vi "Top Menu.vi"(11 "Menu Queue":refnum<queue>) -> ()   [LabVIEW 2013, in "main.lvlib"]
uses:
  main.lvlib
  Controls/Reference AE Control.ctl
  Controls/Reference Cluster.ctl
panel:
  in  "Journal":bool
  in  "Data":bool
  in  "Acquisition":bool
  in  "Configuration":bool
  in  "Profile":bool
  out "PersonalInfoString":string caption="PersonalInfoString2"
  in  "Stop Acq":bool caption="Stop acq"
  in  "MenuStartADC":bool caption="Switch"
  in  "MenuExit":bool caption="Exit"
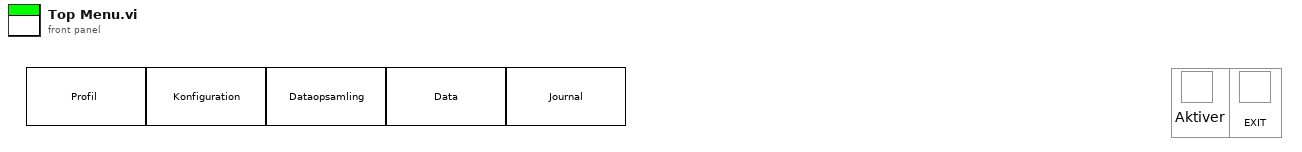
[diagram p1: front panel]
types:
  T1 = typedef "main.lvlib/Reference Cluster.ctl" = cluster{"Menu":cluster{"References":cluster{"Stop Acq":refnum<vi>, "MenuExit":refnum<vi>, "MenuStartADC":refnum<vi>, "PersonalInfoString":refnum<vi>, "Profile":refnum<vi>, "Configuration":refnum<vi>, "Acquisition":refnum<vi>, "Data":refnum<vi>, "Journal":refnum<vi>}}, "Profile":cluster{"References":cluster{"Search Patient ID":refnum<vi>, "Name":refnum<vi>, "CommentStr":refnum<vi>, "Listbox Patient ID":refnum<vi>, "ListboxDoctor":refnum<vi>, "ListboxOperator":refnum<vi>, "HospitalName":refnum<vi>, "HospitalDepartment":refnum<vi>, "HospitalAddress":refnum<vi>, "EditHospInfo":refnum<vi>, "Add Patient ID Btn":refnum<vi>, "Query Worklist":refnum<vi>}}, "Configuration":cluster{"References":cluster{"ListboxMeasurementArea":refnum<vi>, "ListboxMeasurementTechnique":refnum<vi>, "ListboxMeasurementMeth":refnum<vi>, "ListboxRightSegmentNr":refnum<vi>, "ListboxLeftSegmentNr":refnum<vi>, "HeightAdjustmentInt":refnum<vi>, "PalpationRight":refnum<vi>, "PalpationLeft":refnum<vi>, "ActivityBox":refnum<vi>}, "New method":cluster{"AddNewMeasurementBtn":refnum<vi>, "Left Time Table":refnum<vi>, "Right Time Table":refnum<vi>}, "Old method":cluster{"LeftArmPressureTable":refnum<vi>, "RightArmPressureTable":refnum<vi>, "SaveArmPressureBtn":refnum<vi>, "Puls":refnum<vi>, "TempTwo":refnum<vi>, "TempOne":refnum<vi>}, "Method":string}, "Acquisition":cluster{"References":cluster{"SegmentAcqString":refnum<vi>, "RingActGraph":refnum<vi>}}, "Data":cluster{"References":cluster{"cmString":refnum<vi>, "AdjustedHeight":refnum<vi>, "Menu":refnum<vi>, "Tangent On/Off":refnum<vi>, "FilterControl":refnum<vi>}}, "Journal":cluster{"References":cluster{"ReportSelection":refnum<vi>, "Data":refnum<vi>, "GenerateReport":refnum<vi>, "Menu":refnum<vi>, "Send To PACS":refnum<vi>}}}
  T2 = typedef "main.lvlib/Reference AE Control.ctl" = enum16{"Initialize", "Set Menu", "Set Profile", "Set Configuration", "Set Configuration_old", "Set Configuration_new", "Set Configuration Method", "Set Acquisition", "Set Data", "Set Journal", "Get"}
  T3 = cluster{"Stop Acq":refnum<vi>, "MenuExit":refnum<vi>, "MenuStartADC":refnum<vi>, "PersonalInfoString":refnum<vi>, "Profile":refnum<vi>, "Configuration":refnum<vi>, "Acquisition":refnum<vi>, "Data":refnum<vi>, "Journal":refnum<vi>}
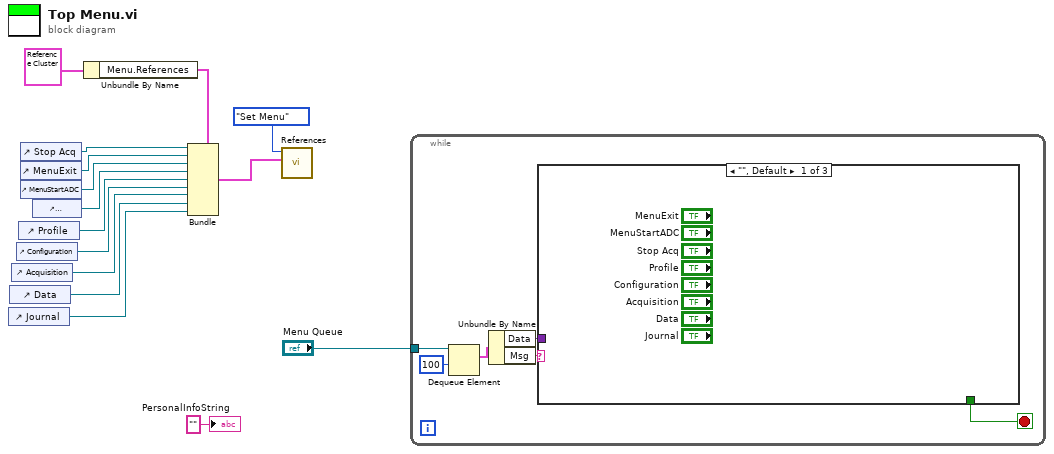
[diagram p0: block diagram]
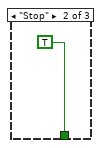
[diagram p2: hidden frame]
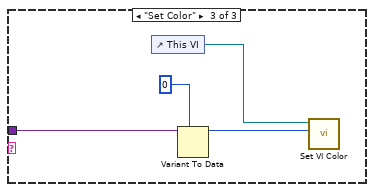
[diagram p3: hidden frame]
diagram:
  n1 = control-ref of="Journal"() -> (w2:refnum<vi>)
  n2 = control-ref of="Data"() -> (w3:refnum<vi>)
  n3 = control-ref of="Acquisition"() -> (w4:refnum<vi>)
  n4 = control-ref of="Configuration"() -> (w5:refnum<vi>)
  n5 = control-ref of="Profile"() -> (w6:refnum<vi>)
  n6 = control-ref of="Stop Acq"() -> (w15:refnum<vi>)
  n7 = control-ref of="MenuExit"() -> (w14:refnum<vi>)
  n8 = control-ref of="MenuStartADC"() -> (w13:refnum<vi>)
  n9 = control-ref of="PersonalInfoString"() -> (w12:refnum<vi>)
  n10 = Unbundle By Name(T1 {"Menu"={"References"={"Stop Acq"=refnum, "MenuExit"=refnum, "MenuStartADC"=refnum, "PersonalInfoString"=refnum, "Profile"=refnum, "Configuration"=refnum, "Acquisition"=refnum, "Data"=refnum, "Journal"=refnum}}, "Profile"={"References"={"Search Patient ID"=refnum, "Name"=refnum, "CommentStr"=refnum, "Listbox Patient ID"=refnum, "ListboxDoctor"=refnum, "ListboxOperator"=refnum, "HospitalName"=refnum, "HospitalDepartment"=refnum, "HospitalAddress"=refnum, "EditHospInfo"=refnum, "Add Patient ID Btn"=refnum, "Query Worklist"=refnum}}, "Configuration"={"References"={"ListboxMeasurementArea"=refnum, "ListboxMeasurementTechnique"=refnum, "ListboxMeasurementMeth"=refnum, "ListboxRightSegmentNr"=refnum, "ListboxLeftSegmentNr"=refnum, "HeightAdjustmentInt"=refnum, "PalpationRight"=refnum, "PalpationLeft"=refnum, "ActivityBox"=refnum}, "New method"={"AddNewMeasurementBtn"=refnum, "Left Time Table"=refnum, "Right Time Table"=refnum}, "Old method"={"LeftArmPressureTable"=refnum, "RightArmPressureTable"=refnum, "SaveArmPressureBtn"=refnum, "Puls"=refnum, "TempTwo"=refnum, "TempOne"=refnum}, "Method"=""}, "Acquisition"={"References"={"SegmentAcqString"=refnum, "RingActGraph"=refnum}}, "Data"={"References"={"cmString"=refnum, "AdjustedHeight"=refnum, "Menu"=refnum, "Tangent On/Off"=refnum, "FilterControl"=refnum}}, "Journal"={"References"={"ReportSelection"=refnum, "Data"=refnum, "GenerateReport"=refnum, "Menu"=refnum, "Send To PACS"=refnum}}} ("Cluster")) -> ("Menu.References"=w8:T3)
  n11 = Bundle(cluster=w8, "Stop Acq"=w15, "MenuExit"=w14, "MenuStartADC"=w13, "PersonalInfoString"=w12, "Profile"=w6, "Configuration"=w5, "Acquisition"=w4, "Data"=w3, "Journal"=w2) -> (w11:T3)
  n12 = call "References.vi"("variant"=w11, "Reference AE Control"=Reference_AE_Control."Set Menu") -> ()  [unwired: 8 in, 2 out]
  n13 = while {
    tunnel: "Menu Queue" -> [w20]
    stop <- w21 stop-if-true
    n14 = Dequeue Element(queue=w20, timeout in ms (-1)=100) -> (element=w19:cluster{"Msg":string, "Data":variant})  [unwired: 1 in, 3 out]
    n15 = Unbundle By Name(w19) -> ("Data"=w17:variant, "Msg"=w16:string)
    n16 = case shown="\"\", Default" w16 {
      tunnel: [_ TRUE _] -> w21
      tunnel: w17 -> [_ _ w23]
      frame "", Default {
      }
      frame "Stop" {
      }
      frame "Set Color" {
        n17 = control-ref of="This VI"() -> (w26:refnum<vi>)
        n18 = Variant To Data(type=u32 0 ("Pane Color"), Variant=w23) -> (data=w24:u32)  [unwired: 1 in, 1 out]
        n19 = call "Set VI Color.vi"("Pane Color"=w24, "VI in"=w26) -> ()  [unwired: 10 in]
      }
    }
  }
  "PersonalInfoString" <- "" ("PersonalInfoString")
